vi "Stop.vi"(8 "error in (no error)":errorcluster, 11 "Wrapper in":refnum<class "Wrapper.lvclass">) -> (0 "error out":errorcluster, 3 "Wrapper out":refnum<class "Wrapper.lvclass">)   [LabVIEW 2020, in "Wrapped Actor.lvlib" / "Wrapper.lvclass"]
uses:
  Wrapper.lvclass
  Wrapper.lvclass/Wrapper.ctl
  <vilib>/ActorFramework/Message Enqueuer/Message Enqueuer.lvclass/Message Enqueuer.ctl
  <vilib>/ActorFramework/Message Enqueuer/Enqueue.vi
  <vilib>/ActorFramework/Stop Msg/Stop Msg.lvclass
  C:/Program Files/National Instruments/LabVIEW 2020/vi.lib/ActorFramework/Message/Message.lvclass
  Actor Pub Sub Channels/Pub Sub Event Channel/Pub Sub Event Channel.lvclass
  E:/Labview/LV 2020/Libs/Actor Pub Sub/Source/Actor Pub Sub Channels/Pub Sub Message Channel/Pub Sub Message Channel.lvclass
  <vilib>/ActorFramework/Message Priority Queue/Priority Enqueue.vi
  Actor Pub Sub Channels/Pub Sub Message Channel/Pub Sub Message Channel.lvclass
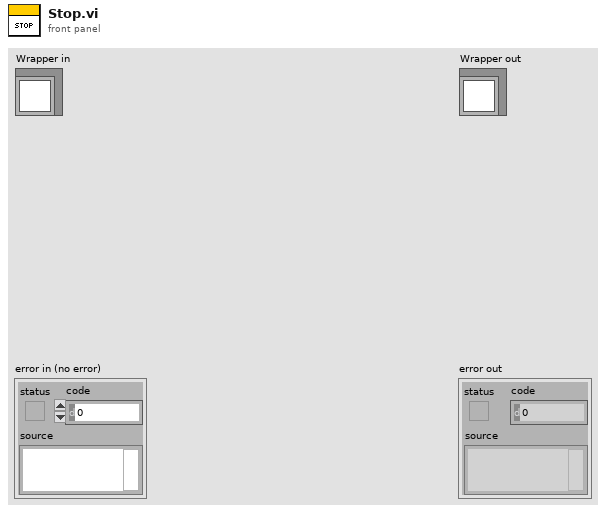
[diagram p1: front panel]
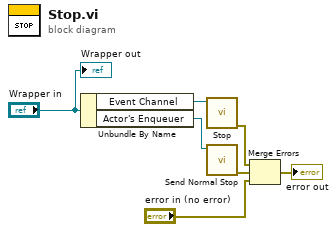
[diagram p0: block diagram]
diagram:
  n1 = Unbundle By Name("Wrapper in") -> ("Event Channel"=w5:refnum<class "Pub Sub Event Channel.lvclass">, "Actor's Enqueuer"=w4:refnum<class "Message Enqueuer.lvclass">)
  n2 = call "Stop.vi"("Pub Sub Message Channel in"=w5) -> ("error out"=w1:errorcluster)  [unwired: 9 in, 1 out]
  n3 = call <vilib>:"Send Normal Stop.vi"("Message Enqueuer"=w4) -> ("error out"=w2:errorcluster)  [unwired: 10 in]
  n4 = Merge Errors(w1, w2, "error in (no error)") -> (→"error out":errorcluster)
  "Wrapper out" <- "Wrapper in"
